vi "Init_Test.vi"(8 "error in (no error)":errorcluster caption="entrée d'erreur (pas d'erreur)", 11 "Stop_Ana IN":refnum<class "Stop_Ana.lvclass">) -> (0 "error out":errorcluster caption="sortie d'erreur", 3 "Stop_Ana Out":refnum<class "Stop_Ana.lvclass">)   [LabVIEW 2020, in "Library Test.lvlib" / "Stop_Ana.lvclass"]
uses:
  Stop_Ana.lvclass
  C:/Users/ngarcin/OneDrive - Altyor/Standard TB/Class/Test/Test (Default)/Test (Default).lvclass
  Commun VI/TypeDef/Commande Test/Commande Value Type.ctl
  Commun VI/TypeDef/Commande Test/Commande Type Test.ctl
  Test_Wtih_Instr/Test_With_Inst.lvclass
  Stop_Ana.lvclass/Stop_Ana.ctl
  Commun VI/Library Commun.lvlib
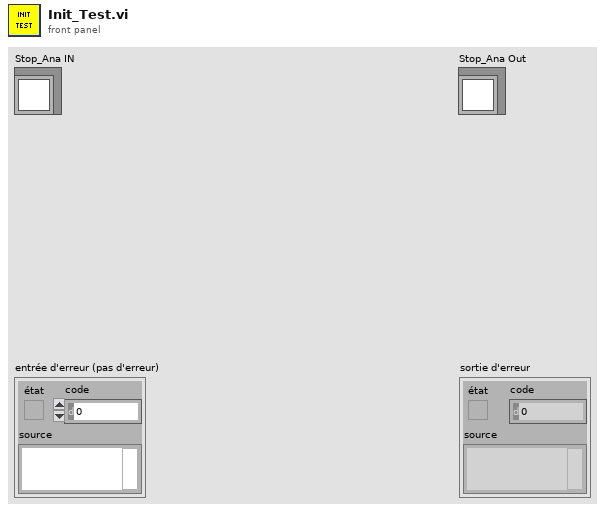
[diagram p1: front panel]
types:
  T1 = typedef "Library Commun.lvlib/Commande Type Test.ctl" = enum16{"Function", "Test", "Calculation"}
  T2 = typedef "Library Commun.lvlib/Commande Value Type.ctl" = enum16{"None", "String", "Number", "Timestamp", "Boolean", "Array"}
  T3 = enum16{"Get Variable", "Get All Variables", "Set Variable", "Delete Variable", "Delete All Variable"}
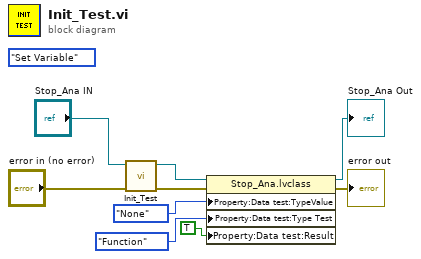
[diagram p0: block diagram]
diagram:
  (unwired) T3."Set Variable" ("Function")
  n1 = call-parent "Init_Test.vi"("error in (no error)"="error in (no error)", "Test_With_Inst en entrée"="Stop_Ana IN") -> ("error out"=w8:errorcluster, "Test_With_Inst en sortie"=w9:refnum<class "Stop_Ana.lvclass">)  [unwired: 8 in]
  n2 = property class="Stop_Ana.lvclass"(reference=w9, error in=w8, "Property:Data test:TypeValue"=Commande_Value_Type."None" ("TypeValue"), "Property:Data test:Type Test"=Commande_Type_Test."Function" ("Type Test"), "Property:Data test:Result"=TRUE ("Result")) -> (reference out=→"Stop_Ana Out":refnum<class "Stop_Ana.lvclass">, error out=→"error out":errorcluster)
